vi "Parse Metadata.vi"(8 "error in":errorcluster, 11 "JSON string (in)":string) -> (0 "error out":errorcluster, 3 "Internal Vars":T1={"Test_File"="", "Status"="Done", "RF_Center_Freq"="0", "RF_Gain"="0", "BB_Gain"="0", "Error"="", "file_max"="0", "file_index"="0"})   [LabVIEW 2017]
uses:
  TypeDef/ESC Internal Data Structure (string).ctl
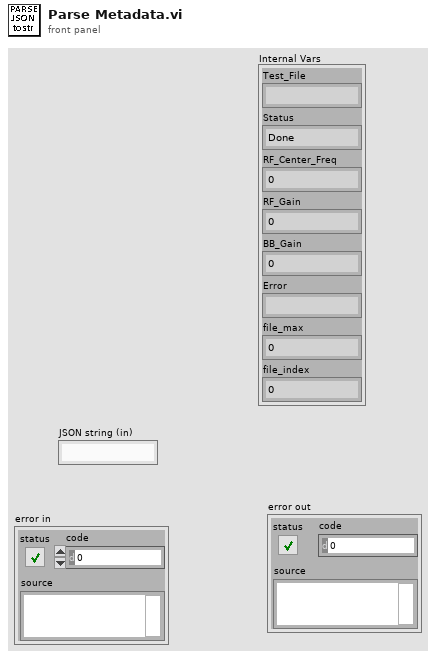
[diagram p1: front panel]
types:
  T1 = typedef "ESC Internal Data Structure (string).ctl" = cluster{"Test_File":string, "Status":string, "RF_Center_Freq":string, "RF_Gain":string, "BB_Gain":string, "Error":string, "file_max":string, "file_index":string}
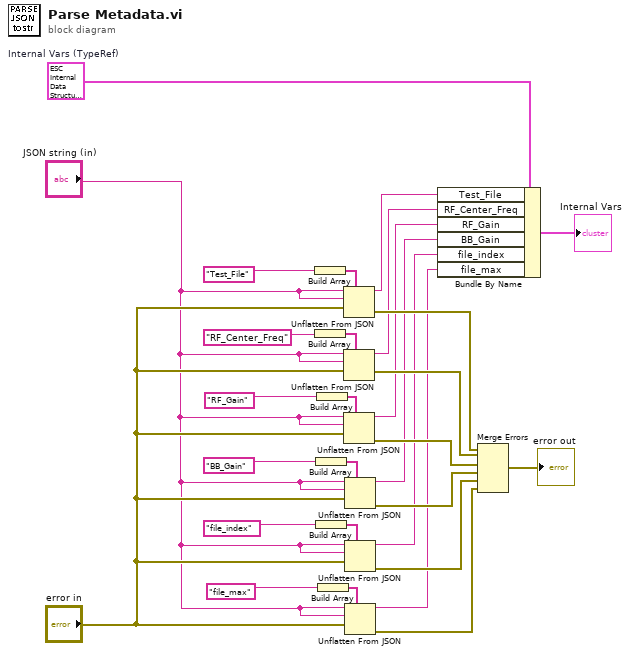
[diagram p0: block diagram]
diagram:
  w4 = T1 {"Test_File"="", "Status"="Done", "RF_Center_Freq"="0", "RF_Gain"="0", "BB_Gain"="0", "Error"="", "file_max"="0", "file_index"="0"}  # Internal Vars (TypeRef)
  n1 = Build Array("Test_File") -> (w28:string[])
  n2 = Build Array("RF_Center_Freq") -> (w26:string[])
  n3 = Build Array("BB_Gain") -> (w22:string[])
  n4 = Build Array("file_index") -> (w20:string[])
  n5 = Build Array("RF_Gain") -> (w24:string[])
  n6 = Build Array("file_max") -> (w18:string[])
  n7 = Unflatten From JSON(path=w28, JSON string="JSON string (in)", type and defaults="JSON string (in)", error in (no error)="error in") -> (value=w10:string, error out=w12:errorcluster)  [unwired: 3 in]
  n8 = Unflatten From JSON(path=w26, JSON string="JSON string (in)", type and defaults="JSON string (in)", error in (no error)="error in") -> (value=w9:string, error out=w13:errorcluster)  [unwired: 3 in]
  n9 = Unflatten From JSON(path=w24, JSON string="JSON string (in)", type and defaults="JSON string (in)", error in (no error)="error in") -> (value=w8:string, error out=w14:errorcluster)  [unwired: 3 in]
  n10 = Unflatten From JSON(path=w22, JSON string="JSON string (in)", type and defaults="JSON string (in)", error in (no error)="error in") -> (value=w11:string, error out=w15:errorcluster)  [unwired: 3 in]
  n11 = Unflatten From JSON(path=w20, JSON string="JSON string (in)", type and defaults="JSON string (in)", error in (no error)="error in") -> (value=w7:string, error out=w16:errorcluster)  [unwired: 3 in]
  n12 = Unflatten From JSON(path=w18, JSON string="JSON string (in)", type and defaults="JSON string (in)", error in (no error)="error in") -> (value=w6:string, error out=w17:errorcluster)  [unwired: 3 in]
  n13 = Bundle By Name(cluster=w4, "Test_File"=w10, "RF_Center_Freq"=w9, "RF_Gain"=w8, "BB_Gain"=w11, "file_index"=w7, "file_max"=w6) -> (→"Internal Vars":T1)
  n14 = Merge Errors(w12, w13, w14, w15, w16, w17) -> (→"error out":errorcluster)
